vi "Begin.vi"(8 "error in":errorcluster) -> (0 "error out":errorcluster)   [LabVIEW 2016]
doc: "Called before other user functions, this VI is expected to open initial I/O refnums, load in file data, and do all program initialization. Notice that the <B>error out</B> terminal is simply used for data flow. Wiring it to other structures or subVIs ensures that this VI runs first."
uses:
  <vilib>/Rock Robotics/SystemInterfaces/DIO/FPGA_DIOPWMChannel.ctl
  <vilib>/Rock Robotics/WPI/SafetyOutput/WPI_SafetyOutputConfigMenu.ctl
  <vilib>/Rock Robotics/WPI/DriverStation/WPI_DriverStationRobotMode2.ctl
  <vilib>/Rock Robotics/WPI/Joystick/WPI_JoystickDeviceEnum.ctl
  Control 6.ctl
  Control 8.ctl
  Control 9.ctl
  Control 13.ctl
  Robot Global Data.vi
  <vilib>/Rock Robotics/WPI/RobotDrive/WPI_RobotDriveOpen2MotorWithTalon.vi
  <vilib>/Rock Robotics/WPI/Solenoid/WPI_SolenoidOpenDouble.vi
  <vilib>/Rock Robotics/WPI/MotorControl/WPI_MotorControlOpen Victor.vi
  <vilib>/Rock Robotics/WPI/Utilities/WPI_GetSetVariantRefNum.vi
  <vilib>/Rock Robotics/WPI/Switch/WPI_SwitchOpenLimit.vi
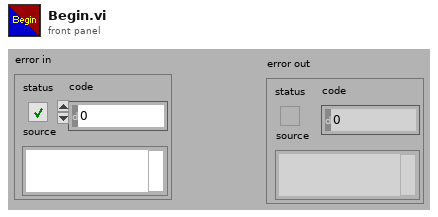
[diagram p1: front panel]
types:
  T1 = typedef "WPI_JoystickDeviceEnum.ctl" = enum16{"USB 0", "USB 1", "USB 2", "USB 3", "USB 4", "USB 5"}
  T2 = typedef "Control 13.ctl" = enum16{"DIO 0", "DIO 1", "DIO 2", "DIO 3", "DIO 4", "DIO 5", "DIO 6", "DIO 7", "DIO 8", "DIO 9"}
  T3 = typedef "Control 6.ctl" = enum16{"Controller 0", "Controller 1", "Controller 2", "Controller 3", "Controller 4", "Controller 5", "Controller 6", "Controller 7"}
  T4 = typedef "Control 9.ctl" = enum16{"Solenoid 0", "Solenoid 1", "Solenoid 2", "Solenoid 3"}
  T5 = typedef "Control 8.ctl" = enum16{"Solenoid 0", "Solenoid 1", "Solenoid 2", "Solenoid 3"}
  T6 = typedef "FPGA_DIOPWMChannel.ctl" = enum8{"PWM 0", "PWM 1", "PWM 2", "PWM 3", "PWM 4", "PWM 5", "PWM 6", "PWM 7", "PWM 8", "PWM 9", "PWM MXP 0", "PWM MXP 1", "PWM MXP 2", "PWM MXP 3", "PWM MXP 4", "PWM MXP 5", "PWM MXP 6", "PWM MXP 7", "PWM MXP 8", "PWM MXP 9", "Invalid"}
  T7 = typedef "WPI_DriverStationRobotMode2.ctl" = enum16{"Autonomous Disabled", "Autonomous Enabled", "Teleop Disabled", "Teleop Enabled", "Disconnected", "Finish", "Test Disabled", "Test Enabled", "Emergency Stopped"}
  T8 = typedef "WPI_SafetyOutputConfigMenu.ctl" = enum16{"Enable", "Disable"}
  T9 = typedef "WPI_JoystickDevRef.ctl" = cluster{"Device":T1}
  T10 = typedef "WPI_CompressorDevRef.ctl" = cluster{"DevStatus":errorcluster, "Pneumatics Control Module":u8}
  T11 = typedef "WPI_RobotDriveDevRef.ctl" = cluster{"DevStatus":errorcluster, "Motors[]":T12[], "Square Inputs":bool, "Max Output":dbl}
  T12 = typedef "WPI_MotorControlDeviceRef.ctl" = cluster{"DeviceStatus":errorcluster, "Type":T13, "PWM":cluster{"PWM Channel":T6, "DeadBand":T14}, "CAN":cluster{"Device Number":u8, "SetOutput VI Ref":variant, "GetOutput VI Ref":variant, "Enable VI Ref":variant, "Disable VI Ref":variant, "Data":variant}, "Invert":bool}
  T13 = typedef "WPI_MotorControlType.ctl" = enum16{"PWM", "CAN"}
  T14 = typedef "WPI_PWMDeadband.ctl" = cluster{"Name":string, "maxPositivePwm":i32, "minPositivePwm":i32, "centerPwm":i32, "maxNegativePwm":i32, "minNegativePwm":i32, "angularRange":u16}
  T15 = typedef "WPI_SwitchDevRef.ctl" = cluster{"DevStatus":errorcluster, "DIO Channel":T16, "CntIndex":T17, "Normally Closed":bool}
  T16 = typedef "FPGA_DIOChannel.ctl" = enum8{"DIO 0", "DIO 1", "DIO 2", "DIO 3", "DIO 4", "DIO 5", "DIO 6", "DIO 7", "DIO 8", "DIO 9", "DIO MXP 0", "DIO MXP 1", "DIO MXP 2", "DIO MXP 3", "DIO MXP 4", "DIO MXP 5", "DIO MXP 6", "DIO MXP 7", "DIO MXP 8", "DIO MXP 9", "DIO MXP 10", "DIO MXP 11", "DIO MXP 12", "DIO MXP 13", "DIO MXP 14", "DIO MXP 15", "SPI Port CS1", "SPI Port CS2", "SPI Port CS3", "SPI Port MISO", "SPI Port MOSI", "Invalid"}
  T17 = typedef "FPGA_CounterCtrSystemIndex.ctl" = enum8{"Ctr 0", "Ctr 1", "Ctr 2", "Ctr 3", "Ctr 4", "Ctr 5", "Ctr 6", "Ctr 7", "Invalid"}
  T18 = typedef "WPI_SolenoidDevRef.ctl" = cluster{"DevStatus":errorcluster, "Pneumatics Control Module":u8, "Forward Solenoid Channel":T19, "Reverse Solenoid Channel":T19}
  T19 = typedef "WPI_SolenoidChannel.ctl" = enum8{"Solenoid 0", "Solenoid 1", "Solenoid 2", "Solenoid 3", "Solenoid 4", "Solenoid 5", "Solenoid 6", "Solenoid 7", "Invalid"}
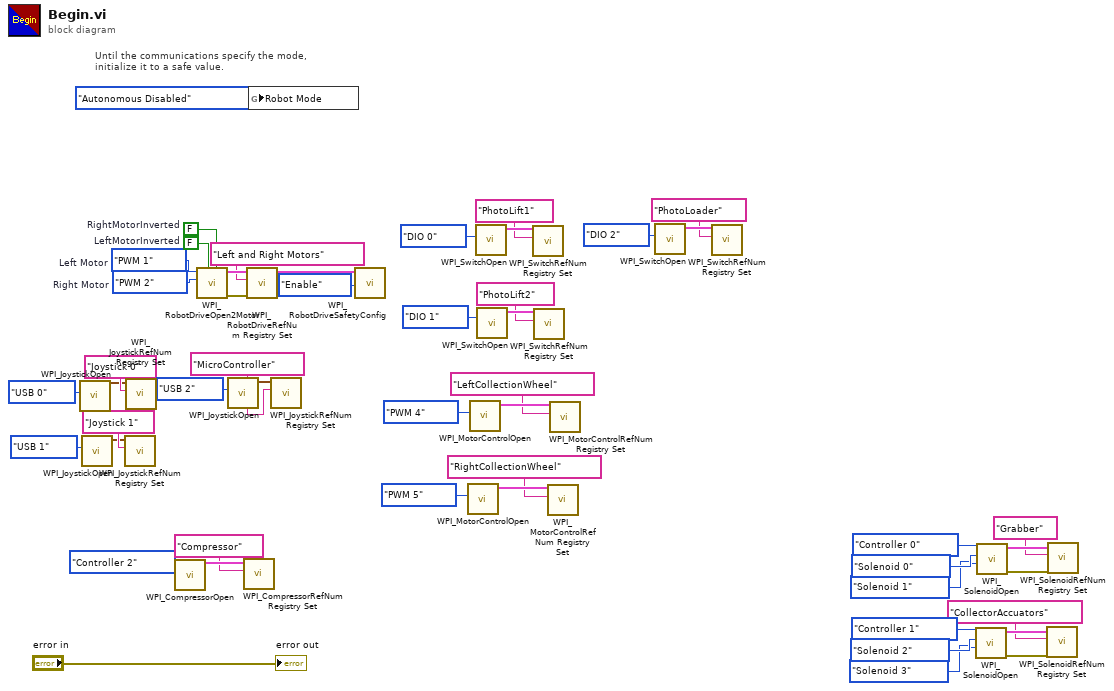
[diagram p0: block diagram]
diagram:
  w37 = FPGA_DIOPWMChannel."PWM 2"  # Right Motor
  w38 = FPGA_DIOPWMChannel."PWM 1"  # Left Motor
  w49 = FALSE  # LeftMotorInverted
  w50 = FALSE  # RightMotorInverted
  # "Until the communications specify the mode,\ninitialize it to a safe value."
  n1 = call <vilib>:"WPI_JoystickOpen.vi"("JoystickDevice"=WPI_JoystickDeviceEnum."USB 0") -> ("JoystickDevRef"=w35:T9)  [unwired: 10 in]
  n2 = call <vilib>:"WPI_JoystickOpen.vi"("JoystickDevice"=WPI_JoystickDeviceEnum."USB 1") -> ("JoystickDevRef"=w41:T9)  [unwired: 10 in]
  n3 = call <vilib>:"WPI_JoystickRefNum Registry Set.vi"("refnum name"="Joystick 1", "JoystickDevRef"=w41) -> ()  [unwired: 8 in, 2 out]
  n4 = call <vilib>:"WPI_JoystickRefNum Registry Set.vi"("refnum name"="Joystick 0", "JoystickDevRef"=w35) -> ()  [unwired: 8 in, 2 out]
  n5 = call <vilib>:"WPI_CompressorOpen.vi"("Pneumatics Control Module (0)"=Control_6."Controller 2") -> ("CompressorDevRef"=w15:T10)  [unwired: 13 in, 1 out]
  n6 = call-poly <vilib>:"WPI_RobotDriveOpen2Motor.vi"("Right Motor Inverted"=w50, "Left Motor Inverted"=w49, "Right Motor"=w37, "Left Motor"=w38) -> ("error out"=w46:errorcluster, "RobotDriveDevRef"=w48:T11)  [unwired: 6 in]
  n7 = call <vilib>:"WPI_JoystickOpen.vi"("JoystickDevice"=WPI_JoystickDeviceEnum."USB 2") -> ("JoystickDevRef"=w2:T9)  [unwired: 10 in]
  n8 = call <vilib>:"WPI_CompressorRefNum Registry Set.vi"("refnum name"="Compressor", "CompressorDevRef"=w15) -> ()  [unwired: 8 in, 2 out]
  n9 = call <vilib>:"WPI_RobotDriveRefNum Registry Set.vi"("error in (no error)"=w46, "refnum name"="Left and Right Motors", "RobotDriveDevRef"=w48) -> ("RobotDriveDevRef"=w45:T11)  [unwired: 1 in, 7 out]
  n10 = global write "Robot Global Data.vi" "Robot Mode"(WPI_DriverStationRobotMode2."Autonomous Disabled" ("Robot Mode")) -> ()
  n11 = call <vilib>:"WPI_JoystickRefNum Registry Set.vi"("refnum name"="MicroController", "JoystickDevRef"=w2) -> ()  [unwired: 8 in, 2 out]
  n12 = call <vilib>:"WPI_RobotDriveSafetyConfig.vi"("mode"=WPI_SafetyOutputConfigMenu."Enable", "RobotDriveDevRef"=w45) -> ()  [unwired: 8 in, 2 out]
  n13 = call-poly <vilib>:"WPI_MotorControlOpen.vi"("PWM Channel"=FPGA_DIOPWMChannel."PWM 5") -> ("MotorControlDeviceRef"=w24:T12)  [unwired: 9 in, 1 out]
  n14 = call-poly <vilib>:"WPI_MotorControlOpen.vi"("PWM Channel"=FPGA_DIOPWMChannel."PWM 4") -> ("MotorControlDeviceRef"=w27:T12)  [unwired: 9 in, 1 out]
  n15 = call-poly <vilib>:"WPI_SwitchOpen.vi"("DIO Channel"=Control_13."DIO 0") -> ("SwitchDevRef"=w12:T15)  [unwired: 9 in, 1 out]
  n16 = call-poly <vilib>:"WPI_SwitchOpen.vi"("DIO Channel"=Control_13."DIO 1") -> ("SwitchDevRef"=w10:T15)  [unwired: 9 in, 1 out]
  n17 = call <vilib>:"WPI_SwitchRefNum Registry Set.vi"("refnum name"="PhotoLift1", "SwitchDevRef"=w12) -> ()  [unwired: 8 in, 2 out]
  n18 = call <vilib>:"WPI_SwitchRefNum Registry Set.vi"("refnum name"="PhotoLift2", "SwitchDevRef"=w10) -> ()  [unwired: 8 in, 2 out]
  n19 = call <vilib>:"WPI_MotorControlRefNum Registry Set.vi"("refnum name"="RightCollectionWheel", "MotorControlDevRef"=w24) -> ()  [unwired: 8 in, 2 out]
  n20 = call <vilib>:"WPI_MotorControlRefNum Registry Set.vi"("refnum name"="LeftCollectionWheel", "MotorControlDevRef"=w27) -> ()  [unwired: 8 in, 2 out]
  n21 = call-poly <vilib>:"WPI_SwitchOpen.vi"("DIO Channel"=Control_13."DIO 2") -> ("SwitchDevRef"=w8:T15)  [unwired: 9 in, 1 out]
  n22 = call <vilib>:"WPI_SwitchRefNum Registry Set.vi"("refnum name"="PhotoLoader", "SwitchDevRef"=w8) -> ()  [unwired: 8 in, 2 out]
  n23 = call-poly <vilib>:"WPI_SolenoidOpen.vi"("Reverse Solenoid Channel"=Control_9."Solenoid 3", "Forward Solenoid Channel"=Control_8."Solenoid 2", "Pneumatics Control Module (0)"=Control_6."Controller 1") -> ("error out"=w19:errorcluster, "SolenoidDevRef"=w21:T18)  [unwired: 7 in]
  n24 = call-poly <vilib>:"WPI_SolenoidOpen.vi"("Reverse Solenoid Channel"=Control_9."Solenoid 1", "Forward Solenoid Channel"=Control_8."Solenoid 0", "Pneumatics Control Module (0)"=Control_6."Controller 0") -> ("error out"=w31:errorcluster, "SolenoidDevRef"=w33:T18)  [unwired: 7 in]
  n25 = call <vilib>:"WPI_SolenoidRefNum Registry Set.vi"("error in (no error)"=w19, "refnum name"="CollectorAccuators", "SolenoidDevRef"=w21) -> ()  [unwired: 7 in, 2 out]
  n26 = call <vilib>:"WPI_SolenoidRefNum Registry Set.vi"("error in (no error)"=w31, "refnum name"="Grabber", "SolenoidDevRef"=w33) -> ()  [unwired: 7 in, 2 out]
  "error out" <- "error in"
